vi "Tetra_RX-PROD_Payload.vi"(8 "error in":errorcluster, 10 "Input Constants":string[](array[string]), 11 "Parameters":string[](array[string])=["room", "18.75", "1", "0", "1", "15.5", "31.5"]) -> (0 "error out":errorcluster={"status"=FALSE, "code"=1073676294, "source"="VISA Read in Tetra Loop Serial.vi:4650001->Tetra_Read Imon.vi->Tetra_TX_Payload.vi"}, 2 "Payload Results":string[](array[string])=["0.000", "0.000", "0.000", "0.000", "0.000", "0.000", "0.000", "0.000", "-32.000", "1.000", "18.390", "0.998", "1.810", "3.312", "0.996", "1.198", "5.011", "3.316", "2.513", "2.513", "3.600", "5.496", "2.776", "2.768", "2.280", "1.360", "0.187", "0.089", "0.321", "0.340", "1.483", "0.530", "0.827", "7.000", "P0003", "trace file path"])   [LabVIEW 2018]
uses:
  <vilib>/Utility/error.llb/whitespace.ctl
  86bda725-ccdc-470a-af55-6d3338402ab6.vi
  75c5a050-687e-4f44-8c48-20552f3390b7.vi
  458b4a15-084f-46bd-ad65-8d84519d0715.vi
  e7e3a4d5-9ed6-4285-8f90-f7af1205463a.vi
  778a857b-ea1c-4c41-85f0-8bde546241f8.vi
  765396e5-d7fa-4d1d-a6be-20604e030d46.vi
  498168d9-979f-4171-bbb2-b986919cd012.vi
  fd570da2-80e1-4258-b5ac-03cfe2f2c2d7.vi
  51f53847-2d88-46b1-9baf-ea88b261c08d.vi
  7f90040b-45cf-45e9-9a76-a1a76b3da838.vi
  Initialize References/Station References Global.vi
  Initialize References/Sequence Globals.vi
  Tetra_Globals.vi
  Infrastructure/Test Result File Name Global.vi
  Infrastructure/Test Parameter Globals_1.0.0.vi
  Instruments/Agilent N5232A PNA-L/Labview Driver/Keysight PNA Series/Keysight PNA Series.lvlib
  Instruments/PNA/lib functions/Agilent ENA Series.lvlib
panel:
  out "#of_adc-resyncs":i32
  out "result path":string
  out "ser_rd":string
  out "readback":string
  out "NF_OFS_GHZ":dbl
  out "RX-PASS?(T)":bool
  out "no_fault":bool
  out "FH_NOT(T)":bool
  in  "ess_error":errorcluster
  out "STOP(T)":bool
  in  "Tab Control":enum32{"Page 1", "Page 2", "Page 3", "Page 4"}(tab)
  out "MEAS_DCMON":bool=TRUE
  out "MEAS_ADAR_TEMP":bool
  out "MEAS_PLATE_TEMP":bool
  out "MODE":bool
  out "ADC_ETH(T)":bool
  out "ADC_CAL(t)":bool
  out "ADC_SYNC_NOT":bool
  out "dBFS_REF":dbl
  out "#OFAVGs-Sig":i32
  out "Temp Soak(min)":dbl
  out "NF Freq Out":dbl
  out "RX_GAIN(t)":bool
  out "RX_FILT(t)":bool
  out "RF_POWER(t)":bool
  out "RX_PORT(t)":bool
  out "V_SUPPLY(t)":bool
  out "TEMP(t)":bool
  out "REF_PWR(t)":bool
  out "RF_FREQ(t)":bool
  out "ref_freq(t)":bool
  out "freq/filt change":bool
  out "MEAS_PS":bool=TRUE
  out "GET_TRACE":bool
  out "MEAS_SNR":bool
  out "TEMP":dbl
  out "RX_PORT":i32
  out "REF_POW":dbl=1.0
  out "V_SUPPLY":dbl=18.75
  out "RF_POWER":dbl=6.0
  out "RX_FILT":i32=32
  out "RX_GAIN":i32
  out "RF_FREQ":dbl
  out "GAIN_HSL":dbl
  out "GAIN_LSL":dbl
  out "NF_LSL":dbl
  out "adc_lock(t)":bool
  out "freq_lock(t)":bool
  out "NF_HSL":dbl
  out "RunAM_Init":bool=TRUE
  out "rx_gain_auto(t)":bool
  out "rdiv(v)":dbl[](array[numeric])=[3.6, 5.496, 2.776, 2.768, 2.28, 1.36]
  out "rdiv(i)":dbl[](array[numeric])=[0.187, 0.089, 0.321, 0.34, 1.483, 0.53]
  out "rdv":dbl[](array[numeric])=[18.39, 0.998, 1.81, 3.312, 0.996, 1.198, 5.011, 3.316, 2.513, 2.513]
  out "temp_sense1-2":dbl[](array[numeric])
  out "ob_temp":sgl[](array[numeric])
  out "ps_meas(i)(w)":dbl[](array[numeric])
  out "rxgain (1-4)":i32[](array[numeric])
  out "rxpeak_mhz":dbl
  out "rxpeak_dbm":dbl
  out "fout_bp":dbl
  out "rx_bpower_on":dbl
  out "rx_bpower_off":dbl
  out "BW(MHz)":dbl
  out "rx_filt":i32
  out "bpf":i32=1
  out "noisecapture path":string
  out "sigcapture path":string
  out "TraceFilePath":path
  out "DC_LSL":dbl
  out "DC_HSL":dbl
  out "cal_rf_ampl":dbl
  out "cal_ref_ampl":dbl
  out "cal_ref_freq":dbl
  out "cal_rf_freq":dbl
  out "peak_gain":dbl
  out "s-n":dbl
  out "nf":dbl
  out "if_freq":dbl
  out "ref_freq":dbl
  out "Cutoff Freq (GHz)":dbl
  out "adc#ofresync":i32
  out "cal_adc_delay":string
  out "comport":refnum<visa-resource-name>
  out "CalFileA":path
  out "adc_chan_id":string
  out "relative seconds":dbl=73640.4138221 format="%_19f"
  out "ref_cal":dbl[][](array[numeric])
  out "rf_cal":dbl[][](array[numeric])
  out "iteration Time(s)":dbl
  out "#OFAVGs-Noi":i32
  out "NF_MASK":dbl[][](array[numeric])
  out "adcsync":string="rd rxm 0x31\r\n0x031: 0x67\r\n>"
  # "Globals (last value change)"
  # "Vmon & Imon"
  # "Temp Sensors"
types:
  T1 = typedef "whitespace.ctl" = u16
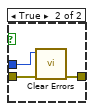
[diagram p3: hidden frame]
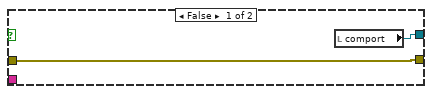
[diagram p4: hidden frame]
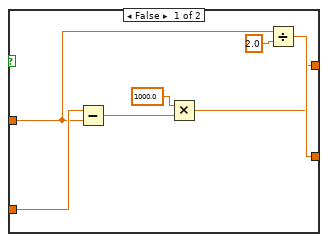
[diagram p5: hidden frame]
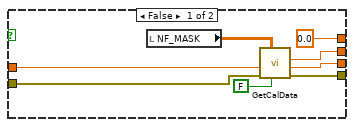
[diagram p7: hidden frame]
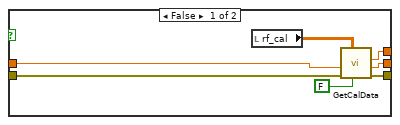
[diagram p8: hidden frame]
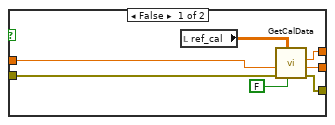
[diagram p9: hidden frame]
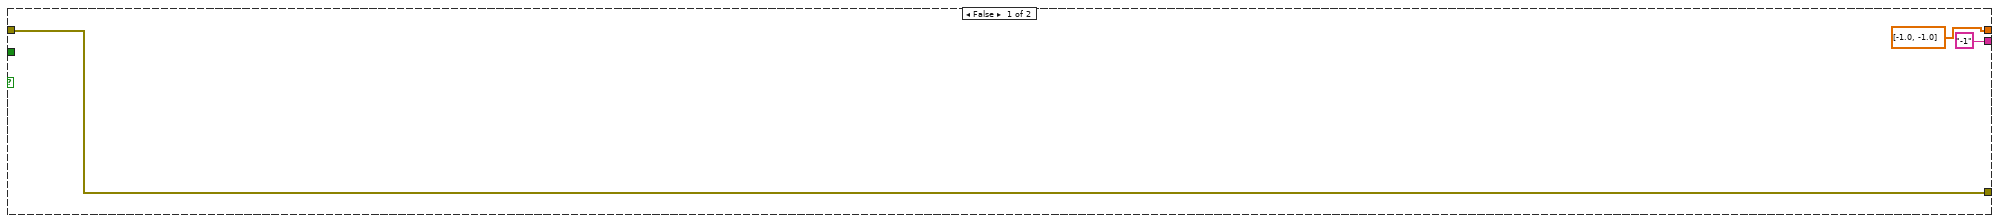
[diagram p11: hidden frame]
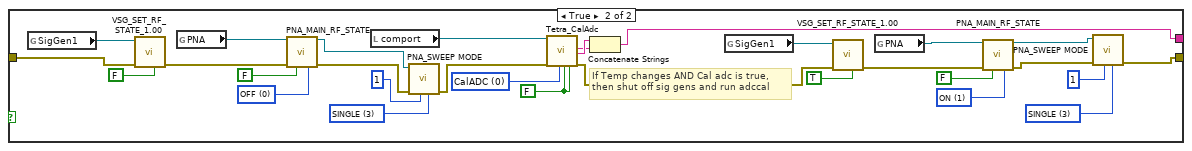
[diagram p12: hidden frame]
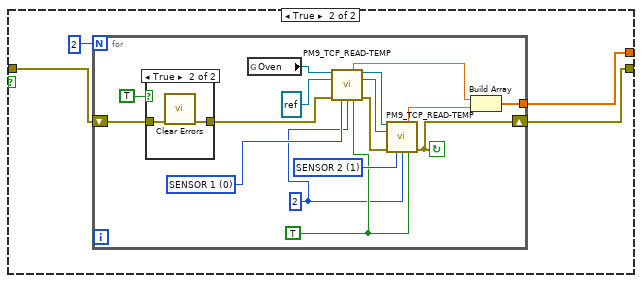
[diagram p13: hidden frame]
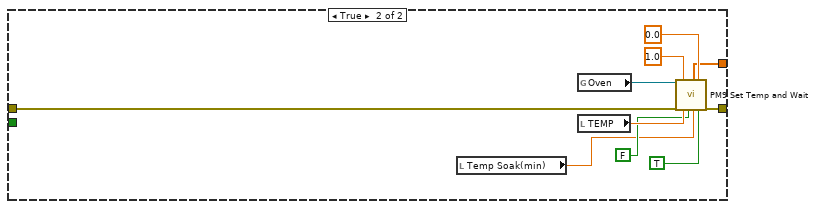
[diagram p15: hidden frame]
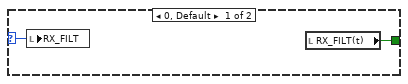
[diagram p16: hidden frame]
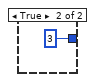
[diagram p17: hidden frame]
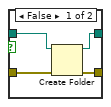
[diagram p19: hidden frame]
diagram:
  n1 = flat-sequence {
    tunnel: [w30] -> w19
    tunnel: [w31] -> w15
    tunnel: "error in" -> [w30]
    tunnel: [w68] -> w29
    tunnel: [w67] -> w28
    tunnel: [w66] -> w27
    tunnel: [w65] -> w26
    tunnel: [w64] -> w25
    tunnel: [w63] -> w24
    tunnel: [w62] -> w23
    tunnel: [w61] -> w22
    tunnel: [w60] -> w21
    tunnel: [w59] -> w20
    tunnel: w19 -> [w58]
    tunnel: [w57] -> w18
    tunnel: [w56] -> w16
    tunnel: w15 -> [w53]
    tunnel: w29 -> [w1117]
    tunnel: w28 -> [w1116]
    tunnel: w27 -> [w1115]
    tunnel: w26 -> [w1114]
    tunnel: w25 -> [w1113]
    tunnel: w24 -> [w1112]
    tunnel: w23 -> [w1111]
    tunnel: w22 -> [w1110]
    tunnel: w21 -> [w1109]
    tunnel: w20 -> [w1108]
    tunnel: w18 -> [w1106]
    tunnel: w16 -> [w1105]
    tunnel: [w1117] -> w13
    tunnel: [w1116] -> w12
    tunnel: [w1115] -> w11
    tunnel: [w1114] -> w10
    tunnel: [w1113] -> w9
    tunnel: [w1112] -> w8
    tunnel: [w1111] -> w7
    tunnel: [w1110] -> w6
    tunnel: [w1109] -> w5
    tunnel: [w1108] -> w4
    tunnel: [w1107] -> w3
    tunnel: [w1106] -> w2
    tunnel: [w1102] -> w1
    tunnel: [w1199] -> w17
    tunnel: w13 -> [w1187]
    tunnel: w12 -> [w1188]
    tunnel: w11 -> [w1189]
    tunnel: w10 -> [w1190]
    tunnel: w9 -> [w1185]
    tunnel: w8 -> [w1184]
    tunnel: w7 -> [w1183]
    tunnel: w6 -> [w1182]
    tunnel: w5 -> [w1186]
    tunnel: w4 -> [w1194]
    tunnel: w3 -> [w1181]
    tunnel: w2 -> [w1199]
    tunnel: w1 -> [w1180]
    frame #0 {
      n2 = flat-sequence {
        frame #0 {
          w49 = TRUE ("Test Running (T)")
          n3 = global read "Station References Global.vi" "Gantry"() -> (w50:refnum<visa-resource-name>)
          n4 = call "WAM_ESS.vi"("VISA resource name"=w50, "error in (no error)"="ess_error", "Open Serial"=w49, "Test Running (T)"=w49, "Close Serial"=w49) -> ("FH_NOT(T)"=→"FH_NOT(T)":bool, "error out"=w47:errorcluster)  [unwired: 7 in, 2 out]
          n5 = local write "ess_error"(w47) -> ()
        }
      }
      n6 = call <vilib>:"High Resolution Relative Seconds.vi"() -> ("relative seconds"=→"relative seconds":dbl)
      n7 = First Call?() -> (First Call?: T/F=w32:bool)
      n8 = case shown="True" w32 {
        frame False {
        }
        frame True {
          (unwired) path "C:/3500007_TetraFinalTestAnalysis/testreport.ini" ("*.ini file")
          n9 = global read "Tetra_Globals.vi" "comport"() -> (w38:refnum<visa-resource-name>)
          n10 = VISA Close(VISA resource name=w38) -> ()  [unwired: 1 in, 1 out]
          n11 = global read "Sequence Globals.vi" "DevSupportPath"() -> (w41:path)
          n12 = global read "Tetra_Globals.vi" "RevC(t)"() -> (w37:bool)
          n13 = global read "Test Result File Name Global.vi" "Test Results File Name"() -> (w36:path)
          n14 = global read "Sequence Globals.vi" "AppSupportPath 2"() -> (w43:path)
          n15 = Not(x=w37) -> ()  [unwired: 1 out]
          n16 = Build Path(base path=w41, name or relative path=path "3500007_TetraFinalTestAnalysis/testreport.ini" ("*.ini file")) -> (appended path=w39:path)
          n17 = Strip Path(path=w39) -> (name=w45:string)  [unwired: 1 out]
          n18 = global read "Sequence Globals.vi" "IsRuntime?"() -> (w44:bool)
          n19 = Build Path(base path=w43, name or relative path=w45) -> (appended path=w42:path)
          n20 = Path To String(path=w36) -> (string=→"result path":string)
          n21 = Select(t=w42, s=w44, f=w39) -> (s? t:f=w46:path)
          n22 = call "ProdLimits.vi"("*.ini file"=w46) -> ()  [unwired: 9 in, 2 out]
          "RunAM_Init" <- TRUE ("RunAM_Init")
        }
      }
      n23 = global read "Sequence Globals.vi" "Stop Testing"() -> (w31:bool)
    }
    frame #1 {
      n24 = Select(t=0, s=w53, f=2) -> (s? t:f=w54:i32)
      n25 = for {
        N: w54 -> [_]
        tunnel: [w95] -> w68
        tunnel: [w94] -> w67
        tunnel: [w93] -> w60
        tunnel: [w92] -> w66
        tunnel: [w91] -> w65
        tunnel: [w90] -> w59
        tunnel: [w89] -> w64
        tunnel: [w88] -> w63
        tunnel: [w87] -> w62
        tunnel: [w86] -> w61
        tunnel: w58 -> [w85]
        shift-right: [w78] -> w57
        shift-left: _ -> [_]
        tunnel: [w72] -> w56 mode=indexing
        i -> [w75]
        stop <- w81 stop-if-true
        n26 = flat-sequence {
          tunnel: [w127] -> w122
          tunnel: ["Parameters"] -> w121
          tunnel: ["Input Constants"] -> w120
          tunnel: w85 -> [w127]
          tunnel: w122 -> [w142]
          tunnel: [w141] -> w119
          tunnel: w121 -> [w212]
          tunnel: w120 -> [w211]
          tunnel: [w203] -> w118
          tunnel: [w199] -> w117
          tunnel: [w210] -> w116
          tunnel: [w209] -> w115
          tunnel: [w208] -> w114
          tunnel: [w187] -> w113
          tunnel: [w207] -> w112
          tunnel: [w200] -> w111
          tunnel: [w189] -> w110
          tunnel: [w161] -> w109
          tunnel: [w175] -> w108
          tunnel: [FALSE] -> w69
          tunnel: w119 -> [w292]
          tunnel: [w292] -> w107
          tunnel: w118 -> [w265]
          tunnel: w117 -> [w289]
          tunnel: w116 -> [w287]
          tunnel: w115 -> [w286]
          tunnel: w114 -> [w284]
          tunnel: w113 -> [w282]
          tunnel: w112 -> [w280]
          tunnel: w111 -> [w276]
          tunnel: w110 -> [w277]
          tunnel: w109 -> [w274]
          tunnel: w108 -> [w271]
          tunnel: w69 -> [w262]
          tunnel: w107 -> [w300]
          tunnel: [w301] -> w106
          tunnel: w106 -> [w366]
          tunnel: [w366] -> w105
          tunnel: [w392] -> w104
          tunnel: w105 -> [w393]
          tunnel: w104 -> [w483]
          tunnel: [w483] -> w103
          tunnel: [w494] -> w82
          tunnel: w103 -> [w493]
          tunnel: [w535] -> w102
          tunnel: w82 -> [w532]
          tunnel: w102 -> [w544]
          tunnel: [w545] -> w101
          tunnel: w101 -> [w564]
          tunnel: [w556] -> w100
          tunnel: w100 -> [w615]
          tunnel: [w614] -> w99
          tunnel: [w705] -> w98
          tunnel: w99 -> [w704]
          tunnel: w98 -> [w726]
          tunnel: [w721] -> w97
          tunnel: w97 -> [w959]
          tunnel: [w958] -> w96
          tunnel: w96 -> [w980]
          tunnel: [w982] -> w84
          tunnel: w84 -> [w1008]
          tunnel: [w1008] -> w71
          tunnel: [w1007] -> w83
          tunnel: w71 -> [w1035]
          tunnel: [w1035] -> w70
          tunnel: [w1048] -> w77
          tunnel: [w1087] -> w95
          tunnel: [w1078] -> w94
          tunnel: [w1082] -> w93
          tunnel: [w1071] -> w92
          tunnel: [w1068] -> w91
          tunnel: [w1063] -> w90
          tunnel: [w1058] -> w89
          tunnel: [w1056] -> w88
          tunnel: [w1053] -> w87
          tunnel: [w1050] -> w86
          tunnel: w70 -> [w1048]
          frame #0 {
          }
          frame #1 {
            n27 = Index Array(array=w211, index #1=2 ("index"), index #2=5 ("index"), index #3=3 ("index"), index #4=6 ("index"), index #6=10 ("index"), index #7=15 ("index"), index #8=13 ("index"), index #9=11 ("index"), index #10=8 ("index"), index #12=18 ("index"), index #13=20 ("index"), index #17=26 ("index")) -> (element #1=w144:string, element #2=w171:string, element #3=w177:string, element #4=w227:string, element #5=w226:string, element #6=w217:string, element #7=w214:string, element #8=w139:string, element #9=w197:string, element #10=w178:string, element #11=w183:string, element #12=w152:string, element #13=w162:string, element #14=w160:string, element #15=w158:string, element #16=w156:string, element #17=→"ser_rd":string)  [unwired: 5 in]
            n28 = call "StringToNumberControlWithBool.vi"("String In"=w177) -> ("NOT = 0"=→"MODE":bool)  [unwired: 7 in, 1 out]
            n29 = call "StringToNumberControlWithBool.vi"("String In"=w227) -> ("Number Out"=→"Temp Soak(min)":dbl)  [unwired: 7 in, 1 out]
            n30 = call "StringToNumberControlWithBool.vi"("String In"=w217) -> ("NOT = 0"=→"GET_TRACE":bool)  [unwired: 7 in, 1 out]
            n31 = Fract/Exp String To Number(string=w197) -> (number=→"Cutoff Freq (GHz)":dbl)  [unwired: 3 in, 1 out]
            n32 = call "StringToNumberControlWithBool.vi"("String In"=w162) -> ("NOT = 0"=→"ADC_CAL(t)":bool)  [unwired: 7 in, 1 out]
            n33 = Fract/Exp String To Number(string=w160) -> (number=→"dBFS_REF":dbl)  [unwired: 3 in, 1 out]
            n34 = String To Path(string=w214) -> (path=→"CalFileA":path)
            n35 = Match Pattern(string=w226, regular expression=";") -> (before substring=w225:string, after substring=w224:string)  [unwired: 1 in, 2 out]
            n36 = call "StringToNumberControlWithBool(x2).vi"("Seperator"=";", "string"=w139) -> ("Num"=→"#OFAVGs-Sig":dbl, "after substring"=w137:string, "Seperator Out"=w134:string)  [unwired: 3 in, 4 out]
            n37 = Match Pattern(string=w178, regular expression=";") -> (before substring=w193:string, after substring=w191:string)  [unwired: 1 in, 2 out]
            n38 = Match Pattern(string=w171, regular expression=";") -> (before substring=w173:string, after substring=w170:string)  [unwired: 1 in, 2 out]
            n39 = Match Pattern(string=w183, regular expression=";") -> (before substring=w182:string, after substring=w181:string)  [unwired: 1 in, 2 out]
            n40 = call "StringToNumberControlWithBool(x2).vi"("Seperator"=";", "string"=w152) -> ("Num(2)"=→"#of_adc-resyncs":dbl, "NOT_0(2)"=w151:bool, "NOT_0?"=→"ADC_ETH(T)":bool, "Seperator Out"=w155:string)  [unwired: 3 in, 3 out]
            n41 = First Call?() -> (First Call?: T/F=w143:bool)
            n42 = Not(x=w151) -> (.not. x?=→"ADC_SYNC_NOT":bool)
            n43 = case shown="True" w143 {
              tunnel: [w231 w237] -> w145
              tunnel: w144 -> [_ w239]
              tunnel: w142 -> [w230 w232]
              tunnel: [w230 w236] -> w141
              frame False {
                n44 = local read "comport"() -> (w231:refnum<visa-resource-name>)
              }
              frame True {
                n45 = Empty String/Path?(string/path=w239) -> (empty?=w240:bool)
                n46 = global read "Tetra_Globals.vi" "comport"() -> (w234:refnum<visa-resource-name>)
                n47 = Select(t=w234, s=w240, f=w239) -> (s? t:f=w238:refnum<visa-resource-name>)
                n48 = call "Tetra Serial.vi"("COMPORT"=w238, "ClearErrorIn(t)"=TRUE, "error in (no error)"=w232, "Open Ser(t)"=TRUE) -> ("comport"=w237:refnum<visa-resource-name>, "error out"=w236:errorcluster)  [unwired: 7 in, 3 out]
              }
            }
            "comport" <- w145
            n49 = call "StringToNumberControlWithBool.vi"("String In"=w225) -> ("NOT = 0"=→"MEAS_PS":bool)  [unwired: 7 in, 1 out]
            n50 = call "StringToNumberControlWithBool.vi"("String In"=w224) -> ("NOT = 0"=→"MEAS_DCMON":bool)  [unwired: 7 in, 1 out]
            n51 = call "StringToNumberControlWithBool(x2).vi"("Seperator"=w134, "string"=w137) -> ("Num(2)"=→"NF_OFS_GHZ":dbl, "Num"=→"#OFAVGs-Noi":dbl)  [unwired: 3 in, 5 out]
            n52 = call "StringToNumberControlWithBool.vi"("String In"=w193) -> ("NOT = 0"=w175:bool)  [unwired: 7 in, 1 out]
            "MEAS_SNR" <- w175
            n53 = call "StringToNumberControlWithBool.vi"("String In"=w191) -> ("Number Out"=→"BW(MHz)":dbl)  [unwired: 7 in, 1 out]
            n54 = Fract/Exp String To Number(string=w170) -> (number=w169:dbl)  [unwired: 3 in, 1 out]
            n55 = Index Array(array=w212) -> (element #1=w187:string, element #2=w220:string, element #3=w219:string, element #4=w206:string, element #5=w205:string, element #6=w195:string, element #7=w204:string, element #8=w202:string)  [unwired: 8 in]
            n56 = call "StringToNumberControlWithBool.vi"("String In"=w182) -> ("NOT = 0"=→"MEAS_ADAR_TEMP":bool)  [unwired: 7 in, 1 out]
            n57 = call "StringToNumberControlWithBool.vi"("String In"=w181) -> ("NOT = 0"=→"MEAS_PLATE_TEMP":bool)  [unwired: 7 in, 1 out]
            n58 = call "StringToNumberControlWithBool(x2).vi"("Seperator"=w155, "string"=w158) -> ("Num(2)"=→"DC_HSL":dbl, "Num"=→"DC_LSL":dbl, "Seperator Out"=w157:string)  [unwired: 3 in, 4 out]
            n59 = Equal?(x=w173, y="fixed") -> (x = y?=w168:bool)
            n60 = call "StringToNumberControlWithBool(x2).vi"("Seperator"=w157, "string"=w156) -> ("Num(2)"=→"GAIN_HSL":dbl, "Num"=→"GAIN_LSL":dbl)  [unwired: 3 in, 5 out]
            n61 = Fract/Exp String To Number(string=w220) -> (number=w208:dbl)  [unwired: 3 in, 1 out]
            "V_SUPPLY" <- w208
            n62 = Decimal String To Number(string=w219) -> (number=w209:i32)  [unwired: 2 in, 1 out]
            "RX_PORT" <- w209
            n63 = Fract/Exp String To Number(string=w206) -> (number=w207:dbl)  [unwired: 3 in, 1 out]
            "REF_POW" <- w207
            n64 = Fract/Exp String To Number(string=w205) -> (number=w210:dbl)  [unwired: 3 in, 1 out]
            "RF_POWER" <- w210
            n65 = Decimal String To Number(string=w195) -> (number=w199:i32)  [unwired: 2 in, 1 out]
            "RX_FILT" <- w199
            n66 = Decimal String To Number(string=w204) -> (number=w203:i32)  [unwired: 2 in, 1 out]
            "RX_GAIN" <- w203
            n67 = call "TempControlWithBool.vi"("INPUT"=w187) -> ("out"=→"TEMP":dbl, "Valid(t)"=w161:bool)  [unwired: 6 in, 1 out]
            n68 = Fract/Exp String To Number(string=w202) -> (number=w200:dbl)  [unwired: 3 in, 1 out]
            "RF_FREQ" <- w200
            n69 = case "calculate the if and ref" shown="True" w168 {
              tunnel: w200 -> [w245 w257]
              tunnel: [w246 w256] -> w189
              tunnel: [w242 w255] -> w188
              tunnel: w169 -> [w244 w248]
              frame False {
                n70 = Subtract(x=w245, y=w244) -> (x-y=w243:dbl)
                n71 = Multiply(x=1000.0, y=w243) -> (x*y=w242:dbl)
                n72 = Divide(x=w244, y=2.0) -> (x/y=w246:dbl)
              }
              frame True {
                w250 = 2.0 ("y")
                n73 = Less Than 0?(x=w248) -> (x < 0?=w249:bool)
                n74 = Divide(x=w248, y=1000.0) -> (x/y=w253:dbl)
                n75 = case shown="True" w249 {
                  tunnel: [w258 w261] -> w255
                  tunnel: w248 -> [w258 w260]
                  frame False {
                  }
                  frame True {
                    n76 = Multiply(x=w260, y=-1.0) -> (x*y=w261:dbl)
                  }
                }
                n77 = Divide(x=w253, y=w250) -> (x/y=w251:dbl)
                n78 = Divide(x=w257, y=w250) -> (x/y=w252:dbl)
                n79 = Add(x=w252, y=w251) -> (x+y=w256:dbl)
              }
            }
            "ref_freq" <- w189
            "if_freq" <- w188
            n80 = global write "Tetra_Globals.vi" "TEMP(t)"(w161) -> ()
          }
          frame #2 {
            # "Check if value changed\nif value changed (t) use to skip the routine"
            n81 = Stop(stop? (T)=w262) -> ()
            n82 = global read "Tetra_Globals.vi" "RX_N_FREQ_LIST"() -> (w269:dbl[])
            n83 = call "Is Value Changed.vim"("value"=w282) -> ("changed or first call?"=w283:bool)
            n84 = call "Is Value Changed.vim"("value"=w277) -> ("changed or first call?"=→"ref_freq(t)":bool)
            n85 = call "Is Value Changed.vim"("value"=w284) -> ("changed or first call?"=→"V_SUPPLY(t)":bool)
            n86 = call "Is Value Changed.vim"("value"=w286) -> ("changed or first call?"=→"RX_PORT(t)":bool)
            n87 = call "Is Value Changed.vim"("value"=w280) -> ("changed or first call?"=→"REF_PWR(t)":bool)
            n88 = call "Is Value Changed.vim"("value"=w287) -> ("changed or first call?"=→"RF_POWER(t)":bool)
            n89 = call "Is Value Changed.vim"("value"=w289) -> ("changed or first call?"=→"RX_FILT(t)":bool)
            n90 = call "Is Value Changed.vim"("value"=w265) -> ("changed or first call?"=→"RX_GAIN(t)":bool)
            n91 = call "Is Value Changed.vim"("value"=w276) -> ("changed or first call?"=→"RF_FREQ(t)":bool)
            n92 = Equal?(x=w265, y=-1) -> (x = y?=→"rx_gain_auto(t)":bool)
            n93 = And(x=w283, y=w274) -> (x .and. y?=→"TEMP(t)":bool)
            n94 = Empty Array?(array=w269) -> (empty?=w267:bool)
            n95 = Array Size(array=w269) -> (size(s)=w273:i32)
            n96 = for {
              tunnel: w269 -> [w299] mode=indexing
              tunnel: [w297] -> w272
              tunnel: w273 -> [w293]
              i -> [w294]
              stop <- w296 stop-if-true
              n97 = local read "RF_FREQ"() -> (w298:dbl)
              n98 = Equal?(x=w293, y=w294) -> (x = y?=w295:bool)
              n99 = Equal?(x=w299, y=w298) -> (x = y?=w297:bool)
              n100 = Or(x=w297, y=w295) -> (x .or. y?=w296:bool)
            }
            n101 = And(x=w272, y=w271) -> (x .and. y?=w270:bool)
            n102 = Or(x=w267, y=w270) -> (x .or. y?=w268:bool)
            n103 = local write "MEAS_SNR"(w268) -> ()
          }
          frame #3 {
            n104 = flat-sequence {
              tunnel: w300 -> [w317]
              tunnel: [w304] -> w301
              frame #0 {
                n105 = local read "ref_freq"() -> (w312:dbl)
                n106 = Multiply(x=1000.0, y=w312) -> (x*y=w310:dbl)
                n107 = First Call?() -> (First Call?: T/F=w309:bool)
                n108 = case shown="True" w309 {
                  tunnel: [w355 w364] -> w319
                  tunnel: [w354 w363] -> w318
                  tunnel: w317 -> [w353 w361]
                  tunnel: [w352 w360] -> w316
                  tunnel: w310 -> [w351 w358]
                  frame False {
                    n109 = local read "ref_cal"() -> (w357:dbl[][])
                    n110 = call "GetCalData.vi"("Open new file T"=FALSE, "Ary In"=w357, "error in (no error)"=w353, "RF Freq (MHz)"=w351) -> ("error out"=w352:errorcluster, "Ampl Out"=w354:dbl, "Cal Freq Out"=w355:dbl)  [unwired: 2 in, 3 out]
                  }
                  frame True {
                    n111 = global read "Tetra_Globals.vi" "REF_CAL"() -> (w365:dbl[][])
                    n112 = call "GetCalData.vi"("Open new file T"=FALSE, "Ary In"=w365, "error in (no error)"=w361, "RF Freq (MHz)"=w358) -> ("error out"=w360:errorcluster, "Ampl Out"=w363:dbl, "Cal Freq Out"=w364:dbl, "array out"=→"ref_cal":dbl[][])  [unwired: 2 in, 2 out]
                  }
                }
                "cal_ref_freq" <- w319
                "cal_ref_ampl" <- w318
                n113 = local read "RF_FREQ"() -> (w302:dbl)
                n114 = Multiply(x=1000.0, y=w302) -> (x*y=w308:dbl)
                n115 = case shown="True" w309 {
                  tunnel: [w340 w349] -> w315
                  tunnel: [w339 w348] -> w314
                  tunnel: w316 -> [w338 w346]
                  tunnel: [w337 w345] -> w305
                  tunnel: w308 -> [w336 w343]
                  frame False {
                    n116 = local read "rf_cal"() -> (w342:dbl[][])
                    n117 = call "GetCalData.vi"("Open new file T"=FALSE, "Ary In"=w342, "error in (no error)"=w338, "RF Freq (MHz)"=w336) -> ("error out"=w337:errorcluster, "Ampl Out"=w339:dbl, "Cal Freq Out"=w340:dbl)  [unwired: 2 in, 3 out]
                  }
                  frame True {
                    n118 = global read "Tetra_Globals.vi" "RX_INPUT_OFFSET"() -> (w350:dbl[][])
                    n119 = call "GetCalData.vi"("Open new file T"=FALSE, "Ary In"=w350, "error in (no error)"=w346, "RF Freq (MHz)"=w343) -> ("error out"=w345:errorcluster, "Ampl Out"=w348:dbl, "Cal Freq Out"=w349:dbl, "array out"=→"rf_cal":dbl[][])  [unwired: 2 in, 2 out]
                  }
                }
                "cal_rf_freq" <- w315
                "cal_rf_ampl" <- w314
                n120 = case shown="True" w309 {
                  tunnel: w302 -> [w327 w334]
                  tunnel: [w326 w333] -> w307
                  tunnel: [0.0 ("NF_LSL") 0.0 ("NF_LSL")] -> w306
                  tunnel: w305 -> [w322 w329]
                  tunnel: [w321 w330] -> w304
                  tunnel: [w320 w328] -> w303
                  frame False {
                    n121 = local read "NF_MASK"() -> (w324:dbl[][])
                    n122 = call "GetCalData.vi"("Open new file T"=FALSE, "Ary In"=w324, "error in (no error)"=w322, "RF Freq (MHz)"=w327) -> ("error out"=w321:errorcluster, "Ampl Out"=w326:dbl, "Cal Freq Out"=w320:dbl)  [unwired: 2 in, 3 out]
                  }
                  frame True {
                    n123 = global read "Tetra_Globals.vi" "NF_MASK"() -> (w335:dbl[][])
                    "NF_MASK" <- w335
                    n124 = call "GetCalData.vi"("Open new file T"=FALSE, "Ary In"=w335, "error in (no error)"=w329, "RF Freq (MHz)"=w334) -> ("error out"=w330:errorcluster, "Ampl Out"=w333:dbl, "Cal Freq Out"=w328:dbl)  [unwired: 2 in, 3 out]
                  }
                }
                "NF_LSL" <- w306
                "NF_HSL" <- w307
                "NF Freq Out" <- w303
              }
            }
          }
          frame #4 {
            n125 = flat-sequence {
              frame #0 {
                n126 = local read "RX_PORT(t)"() -> (w371:bool)
                n127 = local read "ess_error"() -> (w368:errorcluster)
                n128 = And(x=TRUE, y=w371) -> (x .and. y?=w370:bool)
                n129 = case shown="True" w370 {
                  tunnel: w368 -> [w372 w382]
                  tunnel: [w372 w381] -> w367
                  frame False {
                  }
                  frame True {
                    w378 = u16 0 items=["Inches", "cm"] ("Zunits")
                    # "convert to Gantry location"
                    n130 = local read "RX_PORT"() -> (w374:i32)
                    n131 = global read "Tetra_Globals.vi" "Gantry_Z"() -> (w376:dbl)
                    n132 = global read "Station References Global.vi" "Gantry"() -> (w379:refnum<visa-resource-name>)
                    n133 = Subtract(x=21, y=w374) -> (x-y=w373:i32)
                    n134 = call "Gantry.vi"("COMPORT"=w379, "error in (no error)"=w382, "Antenna Select"=w373, "z ref"=21.0, "Write(reads antenna co-ords when off)"=TRUE, "z"=w376, "Zunits"=w378) -> ("error out"=w381:errorcluster)  [unwired: 12 in]
                  }
                }
                n135 = local write "ess_error"(w367) -> ()
              }
            }
          }
          frame #5 {
            n136 = local read "RX_PORT(t)"() -> (w383:bool)
            n137 = local read "MEAS_PLATE_TEMP"() -> (w387:bool)
            n138 = global read "Tetra_Globals.vi" "TEMP(t)"() -> (w390:bool)
            n139 = First Call?() -> (First Call?: T/F=w385:bool)
            n140 = Or(x=w383, y=w385) -> (x .or. y?=w384:bool)
            n141 = Or(x=w390, y=w387) -> (x .or. y?=w389:bool)
            n142 = Or(x=w387, y=w384) -> (x .or. y?=w386:bool)
            n143 = case shown="True" w389 {
              tunnel: w393 -> [w395 w409]
              tunnel: [w395 w403] -> w392
              tunnel: [sgl[] [-1.0, -1.0] ("temp") w408] -> w391
              tunnel: ["-1" ("cal_adc_delay") w400] -> w388
              tunnel: w386 -> [_ w398]
              frame False {
              }
              frame True {
                n144 = global read "Station References Global.vi" "Oven Present?"() -> (w397:bool)
                n145 = local read "ADC_CAL(t)"() -> (w405:bool)
                n146 = local read "TEMP(t)"() -> (w407:bool)
                n147 = And(x=w398, y=w397) -> (x .and. y?=w399:bool)
                n148 = And(x=w407, y=w405) -> (x .and. y?=w406:bool)
                n149 = case shown="False" w407 {
                  tunnel: w409 -> [w445 w477]
                  tunnel: [w443 w476] -> w404
                  tunnel: [w444 w474] -> w408
                  tunnel: w399 -> [w442 _]
                  frame False {
                    n150 = case shown="False" w442 {
                      tunnel: w445 -> [w446 w451]
                      tunnel: [sgl[] [-1.0, -1.0] w450] -> w444
                      tunnel: [w446 w449] -> w443
                      frame False {
                      }
                      frame True {
                        n151 = for {
                          N: 2 -> [_]
                          tunnel: [w462] -> w450
                          shift-right: [w458] -> w449
                          shift-left: w451 -> [w456]
                          stop <- w458 continue-if-true
                          w452 = u32 2 ("milliseconds to wait")
                          w454 = TRUE ("Close tcp(t)")
                          w460 = u16 1 items=["SENSOR 1", "SENSOR 2"] ("Sensor")
                          w461 = u16 0 items=["SENSOR 1", "SENSOR 2"] ("Sensor")
                          n152 = case shown="True" TRUE {
                            tunnel: [w468 w470] -> w457
                            tunnel: w456 -> [w468 w469]
                            frame False {
                            }
                            frame True {
                              n153 = call <vilib>:"Clear Errors.vi"("error in (no error)"=w469) -> ("error out"=w470:errorcluster)  [unwired: 5 in, 1 out]
                            }
                          }
                          n154 = global read "Station References Global.vi" "Oven"() -> (w467:refnum<visa-resource-name>)
                          n155 = call "PM9_TCP_READ-TEMP.vi"("VISA"=w467, "connection ID"=refnum<k5> refnum, "error in (no error)"=w457, "Sensor"=w461, "milliseconds to wait"=w452, "Close tcp(t)"=w454) -> ("Value"=w463:sgl, "visa out"=w459:refnum<visa-resource-name>, "connection ID out"=w466:refnum<k5>, "error out"=w465:errorcluster)  [unwired: 6 in]
                          n156 = call "PM9_TCP_READ-TEMP.vi"("VISA"=w459, "connection ID"=w466, "error in (no error)"=w465, "Sensor"=w460, "milliseconds to wait"=w452, "Close tcp(t)"=w454) -> ("Value"=w464:sgl, "error out"=w458:errorcluster)  [unwired: 6 in, 2 out]
                          n157 = Build Array(w463, w464) -> (w462:sgl[])
                        }
                      }
                    }
                  }
                  frame True {
                    n158 = local read "Temp Soak(min)"() -> (w471:dbl)
                    n159 = global read "Station References Global.vi" "Oven"() -> (w475:refnum<visa-resource-name>)
                    n160 = local read "TEMP"() -> (w473:dbl)
                    n161 = call "PM9 Set Temp and Wait.vi"("VISA"=w475, "Error In"=w477, "Accuracy +/-"=1.0, "Set Point"=w473, "RO(t)"=FALSE, "Min (-1 for cont.)"=w471, "Refresh Rate(s)"=0.0, "close session(t)"=TRUE) -> ("temp"=w474:sgl[], "error out"=w476:errorcluster)  [unwired: 8 in, 2 out]
                  }
                }
                n162 = And(x=FALSE, y=w406) -> (x .and. y?=w402:bool)
                n163 = case shown="False" w402 {
                  tunnel: w404 -> [w411 w440]
                  tunnel: ["-1" ("cal_adc_delay") w415] -> w400
                  tunnel: [w411 w419] -> w403
                  frame False {
                  }
                  frame True {
                    w414 = FALSE ("Open Ser(t)")
                    w418 = 0 items=["CalADC", "ReadADC"] ("ADC_Cal_Function")
                    w431 = 3 items=["HOLD", "CONT", "GROUP", "SINGLE"] ("Mode")
                    w429 = 1 items=["OFF", "ON"] ("STATE(0=OFF)")
                    w432 = 3 items=["HOLD", "CONT", "GROUP", "SINGLE"] ("Mode")
                    w434 = 0 items=["OFF", "ON"] ("STATE(0=OFF)")
                    # "If Temp changes AND Cal adc is true, \nthen shut off sig gens and run adccal"
                    n164 = global read "Station References Global.vi" "SigGen1"() -> (w441:refnum<visa-resource-name>)
                    n165 = call "VSG_SET_RF_STATE_1.00.vi"("RF ON/OFF (OFF)"=FALSE ("Enable RF Power (T: Enable)"), "error in"=w440, "Session In"=w441) -> ("error out"=w439:errorcluster)  [unwired: 6 in, 2 out]
                    n166 = global read "Station References Global.vi" "PNA"() -> (w438:refnum<visa-resource-name>)
                    n167 = call "PNA_MAIN_RF_STATE.vi"("Session In"=w438, "error in"=w439, "RO(T)"=FALSE, "STATE(0=OFF)"=w434) -> ("Session Out"=w437:refnum<visa-resource-name>, "error out"=w436:errorcluster)  [unwired: 9 in, 1 out]
                    n168 = local read "comport"() -> (w413:refnum<visa-resource-name>)
                    n169 = call "PNA_SWEEP MODE.vi"("Mode"=w432, "Channel"=1, "error in (no error)"=w436, "VISA resource name"=w437) -> ("error out"=w412:errorcluster)  [unwired: 6 in, 1 out]
                    n170 = call "Tetra_CalAdc.vi"("COMPORT"=w413, "error in (no error)"=w412, "ADC_Cal_Function"=w418, "Open Ser(t)"=w414, "Close Ser(t)"=w414) -> ("cal_adc_mag"=w416:string, "cal_adc_delay"=w417:string, "error out"=w422:errorcluster)  [unwired: 9 in, 3 out]
                    n171 = Concatenate Strings(w417, w416) -> (w415:string)
                    n172 = global read "Station References Global.vi" "SigGen1"() -> (w423:refnum<visa-resource-name>)
                    n173 = call "VSG_SET_RF_STATE_1.00.vi"("RF ON/OFF (OFF)"=TRUE ("Enable RF Power (T: Enable)"), "error in"=w422, "Session In"=w423) -> ("error out"=w424:errorcluster)  [unwired: 6 in, 2 out]
                    n174 = global read "Station References Global.vi" "PNA"() -> (w425:refnum<visa-resource-name>)
                    n175 = call "PNA_MAIN_RF_STATE.vi"("Session In"=w425, "error in"=w424, "RO(T)"=FALSE, "STATE(0=OFF)"=w429) -> ("Session Out"=w426:refnum<visa-resource-name>, "error out"=w427:errorcluster)  [unwired: 9 in, 1 out]
                    n176 = call "PNA_SWEEP MODE.vi"("Mode"=w431, "Channel"=1, "error in (no error)"=w427, "VISA resource name"=w426) -> ("error out"=w419:errorcluster)  [unwired: 6 in, 1 out]
                  }
                }
              }
            }
            "ob_temp" <- w391
            "cal_adc_delay" <- w388
          }
          frame #6 {
            # "if RX_FILT = -1 then use"
            # "freq driven filter select"
            n177 = local read "RX_FILT"() -> (w481:i32)
            n178 = case shown="-1" w481 {
              selector: w481 -> [w484 _]
              tunnel: [w485 w490] -> w482
              frame 0, Default {
                n179 = local write "RX_FILT"(w484) -> ()
                n180 = local read "RX_FILT(t)"() -> (w485:bool)
              }
              frame -1 {
                n181 = local read "Cutoff Freq (GHz)"() -> (w486:dbl)
                n182 = local read "RF_FREQ"() -> (w487:dbl)
                n183 = Greater Or Equal?(x=w487, y=w486) -> (x >= y?=w489:bool)
                n184 = call "Is Value Changed.vim"("value"=w489) -> ("changed or first call?"=w490:bool)
                n185 = case shown="False" w489 {
                  tunnel: [2 3] -> w488
                  frame False {
                  }
                  frame True {
                  }
                }
                n186 = local write "RX_FILT"(w488) -> ()
              }
            }
            "freq/filt change" <- w482
          }
          frame #7 {
            # "TEMP\nPS1-1_V\nRX_PORT\nREF_POWER\nRF_POWER\nRX_FILT\nRX_GAIN\nRF_FREQ"
            # "Make the path and filename for trace capture"
            n187 = local read "GET_TRACE"() -> (w495:bool)
            n188 = case shown="True" w495 {
              tunnel: [w496 w501] -> w494
              tunnel: w493 -> [w496 w498]
              frame False {
              }
              frame True {
                n189 = local read "Parameters"() -> (w508:string[])
                n190 = global read "Test Result File Name Global.vi" "Test Results File Name"() -> (w512:path)
                n191 = for {
                  tunnel: w508 -> [w527] mode=indexing
                  tunnel: [w525] -> w507 mode=indexing
                  n192 = Concatenate Strings(w527) -> (w526:string)
                  n193 = Search and Replace String(input string=w526, search string=".", replace string="p" ("replace string (\"\")")) -> (result string=w525:string)  [unwired: 5 in, 3 out]
                }
                n194 = Strip Path(path=w512) -> (stripped path=w513:path, name=w516:string)
                n195 = Search and Replace String(input string=w516, search string=".csv", replace string="_RxCaptureFiles" ("name or relative path"), error in=w498) -> (result string=w515:string, error out=w499:errorcluster)  [unwired: 4 in, 2 out]
                n196 = Build Path(base path=w513, name or relative path=w515) -> (appended path=w514:path)
                n197 = Array To Spreadsheet String(delimiter (Tab)="_", array=w507, 3:"%s" ("format string")) -> (spreadsheet string=w509:string)
                n198 = call <vilib>:"Check if File or Folder Exists.vi"("error in (no error)"=w499, "path"=w514) -> ("error out"=w500:errorcluster, "file or folder exists?"=w511:bool)  [unwired: 7 in, 1 out]
                n199 = case shown="True" w511 {
                  tunnel: w514 -> [w522 w524]
                  tunnel: [w521 w524] -> w517
                  tunnel: [w520 w523] -> w501
                  tunnel: w500 -> [w519 w523]
                  frame False {
                    n200 = Create Folder(path (use dialog)=w522, error in=w519) -> (created path=w521:path, error out=w520:errorcluster)  [unwired: 1 in, 1 out]
                  }
                  frame True {
                  }
                }
                n201 = call <vilib>:"Trim Whitespace.vi"("string"=w509) -> ("trimmed string"=w510:string)  [unwired: 1 in]
                n202 = Concatenate Strings(w510, ".csv" ("string")) -> (w518:string)
                n203 = Build Path(base path=w517, name or relative path=w518) -> (appended path=w497:path)
                "TraceFilePath" <- w497
                n204 = global write "Tetra_Globals.vi" "TraceFilePath"(w497) -> ()
              }
            }
          }
          frame #8 {
            # "Set the Power Supply"
            n205 = local read "V_SUPPLY(t)"() -> (w534:bool)
            n206 = local read "RF_FREQ"() -> (w533:dbl)
            n207 = First Call?() -> (First Call?: T/F=w531:bool)
            n208 = local write "RF_FREQ"(w533) -> ()
            n209 = Or(x=w531, y=w534) -> (x .or. y?=w530:bool)
            n210 = case shown="True" w530 {
              tunnel: [w536 w538] -> w535
              tunnel: w532 -> [w536 w537]
              frame False {
              }
              frame True {
                w541 = "PS1"  # SEL_PS
                n211 = local read "V_SUPPLY"() -> (w540:dbl)
                n212 = global read "Station References Global.vi" "PS1"() -> (w542:refnum<visa-resource-name>)
                n213 = call "INST_PS_SET_VOLTAGE_LEVEL_4.0.0.vi"("Instrument Select (Output 1)"="1", "SEL_PS"=w541, "error in (no error)"=w537, "Voltage (0.0)"=w540, "VISA session"=w542) -> ("error out"=w538:errorcluster)  [unwired: 5 in, 1 out]
              }
            }
          }
          frame #9 {
            n214 = local read "MODE"() -> (w543:bool)
            n215 = case shown="True" w543 {
              tunnel: [w546 w552] -> w545
              tunnel: w544 -> [w546 w551]
              frame False {
              }
              frame True {
                w548 = u16 1 items=["MHz", "GHz"] ("Freq Units")
                n216 = local read "comport"() -> (w550:refnum<visa-resource-name>)
                n217 = local read "RF_FREQ"() -> (w549:dbl)
                n218 = call "Tetra_Set-Freq.vi"("COMPORT"=w550, "error in (no error)"=w551, "Freq"=w549, "delay after set(ms)"=u32 10, "Freq Units"=w548) -> ("error out"=w552:errorcluster)  [unwired: 11 in, 3 out]
              }
            }
          }
          frame #10 {
            # "Set the PNA Stimulus"
            n219 = local read "RF_POWER(t)"() -> (w562:bool)
            n220 = case shown="True" w562 {
              tunnel: w564 -> [w592 w594]
              tunnel: [w592 w593] -> w563
              frame False {
              }
              frame True {
                # "Set the RF pow"
                n221 = global read "Station References Global.vi" "SigGen1"() -> (w596:refnum<visa-resource-name>)
                n222 = local read "RF_POWER"() -> (w595:dbl)
                n223 = call "VSG_SET-GET_AMPL_3.00.vi"("error in"=w594, "Set Power (num)"=w595, "Session In"=w596) -> ("error out"=w593:errorcluster)  [unwired: 6 in, 2 out]
              }
            }
            n224 = local read "RF_FREQ(t)"() -> (w565:bool)
            n225 = case shown="True" w565 {
              tunnel: w563 -> [w597 w601]
              tunnel: [w597 w599] -> w558
              frame False {
              }
              frame True {
                # "Set the RF Freq"
                n226 = global read "Station References Global.vi" "SigGen1"() -> (w602:refnum<visa-resource-name>)
                n227 = local read "RF_FREQ"() -> (w600:dbl)
                n228 = call "VSG_SET-GET_CW_1.00.vi"("Freq Units"="GHz", "error in"=w601, "Set Freq (MHz) num"=w600, "Session In"=w602) -> ("error out"=w599:errorcluster)  [unwired: 4 in, 3 out]
              }
            }
            n229 = local read "REF_PWR(t)"() -> (w561:bool)
            n230 = case shown="True" w561 {
              tunnel: w558 -> [w572 w573]
              tunnel: [w572 w576] -> w560
              frame False {
              }
              frame True {
                # "Set the ref pow"
                n231 = global read "Station References Global.vi" "PNA"() -> (w575:refnum<visa-resource-name>)
                n232 = local read "REF_POW"() -> (w579:dbl)
                n233 = call "Select Measurement.vi"("error in (no error)"=w573, "Measurement Name (CH1_S11_1)"="CH1_S11_1", "VISA resource name"=w575) -> ("error out"=w577:errorcluster, "VISA resource name out"=w574:refnum<visa-resource-name>)  [unwired: 7 in]
                n234 = call "Configure Power.vi"("VISA resource name"=w574, "error in (no error)"=w577, "Power Level (0 dBm)"=w579) -> ("error out"=w576:errorcluster)  [unwired: 11 in, 1 out]
              }
            }
            n235 = local read "ref_freq(t)"() -> (w559:bool)
            n236 = case shown="True" w559 {
              tunnel: w560 -> [w580 w585]
              tunnel: [w580 w590] -> w557
              frame False {
              }
              frame True {
                w581 = 1 ("Source")
                w583 = 0 items=["Normal", "SMC"] ("MODE")
                w589 = i64 1000000000 items=["GHz"=1000000000, "MHZ"=1000000] ("Units")
                # "Set the ref Freq"
                n237 = global read "Station References Global.vi" "PNA"() -> (w586:refnum<visa-resource-name>)
                n238 = local read "ref_freq"() -> (w591:dbl)
                n239 = call "Select Measurement.vi"("error in (no error)"=w585, "Measurement Name (CH1_S11_1)"="CH1_S11_1", "Channel (1)"=1, "VISA resource name"=w586) -> ("error out"=w588:errorcluster, "VISA resource name out"=w587:refnum<visa-resource-name>)  [unwired: 6 in]
                n240 = call "PNA-L_SET-CWFREQ.vi"("Session In"=w587, "error in"=w588, "MODE"=w583, "FREQ"=w591, "Units"=w589, "CH"=w581, "Source"=w581) -> ("error out"=w590:errorcluster)  [unwired: 10 in, 2 out]
              }
            }
            n241 = local read "REF_PWR(t)"() -> (w555:bool)
            n242 = local read "ref_freq(t)"() -> (w554:bool)
            n243 = Or(x=w555, y=w554) -> (x .or. y?=w553:bool)
            n244 = case shown="True" w553 {
              tunnel: w557 -> [w566 w570]
              tunnel: [w566 w569] -> w556
              frame False {
              }
              frame True {
                w567 = 3 items=["HOLD", "CONT", "GROUP", "SINGLE"] ("Mode")
                # "take a sweep to make the changes"
                n245 = global read "Station References Global.vi" "PNA"() -> (w571:refnum<visa-resource-name>)
                n246 = call "PNA_SWEEP MODE.vi"("Mode"=w567, "Channel"=1 ("Source"), "error in (no error)"=w570, "VISA resource name"=w571) -> ("error out"=w569:errorcluster)  [unwired: 6 in, 1 out]
              }
            }
          }
          frame #11 {
            # "Set ADAR values"
            n247 = local read "RX_PORT(t)"() -> (w609:bool)
            n248 = case shown="True" w609 {
              tunnel: w615 -> [w685 w689]
              tunnel: [w685 w688] -> w613
              frame False {
              }
              frame True {
                w692 = 0 items=["RX", "TX"] ("RX/TX")
                n249 = local read "RX_PORT"() -> (w691:i32)
                n250 = local read "comport"() -> (w690:refnum<visa-resource-name>)
                n251 = global read "Tetra_Globals.vi" "RevC(t)"() -> (w686:bool)
                n252 = call "Tetra_AntSel.vi"("COMPORT"=w690, "REVC(T)"=w686, "error in (no error)"=w689, "RX/TX"=w692, "ANT(num)"=w691, "milliseconds to wait"=u32 10) -> ("error out"=w688:errorcluster)  [unwired: 11 in, 2 out]
              }
            }
            n253 = local read "freq/filt change"() -> (w612:bool)
            n254 = local read "MODE"() -> (w606:bool)
            n255 = case shown="True" w606 {
              tunnel: w613 -> [w620 w646]
              tunnel: w612 -> [w619 _]
              tunnel: [w618 w641] -> w611
              tunnel: [w617 w645] -> w607
              tunnel: [-1 ("bpf") w636] -> w605
              frame False {
                n256 = case shown="True" w619 {
                  tunnel: w620 -> [w622 w631]
                  tunnel: [w622 w630] -> w618
                  tunnel: [w621 w626] -> w617
                  frame False {
                    n257 = local read "RX_FILT"() -> (w621:i32)
                  }
                  frame True {
                    w628 = 0 items=["RX", "TX"] ("RX/TX")
                    n258 = local read "RX_PORT"() -> (w623:i32)
                    n259 = local read "comport"() -> (w629:refnum<visa-resource-name>)
                    n260 = global read "Tetra_Globals.vi" "RevC(t)"() -> (w624:bool)
                    n261 = local read "RX_FILT"() -> (w625:i32)
                    n262 = call "Tx-RxFilt.vi"("COMPORT"=w629, "REVC(T)"=w624, "AntPort"=w623, "error in (no error)"=w631, "RX/TX"=w628, "VERIFY(t)"=TRUE, "Filt(sel)"=w625) -> ("filt(num)"=w626:i32, "error out"=w630:errorcluster)  [unwired: 10 in, 1 out]
                  }
                }
              }
              frame True {
                w635 = u32 10 ("milliseconds to wait")
                w638 = 0 items=["RX", "TX"] ("RX/TX")
                w643 = 0 items=["RX", "TX"] ("RX/TX")
                n263 = local read "comport"() -> (w644:refnum<visa-resource-name>)
                n264 = global read "Tetra_Globals.vi" "RevC(t)"() -> (w634:bool)
                n265 = local read "RX_PORT"() -> (w633:i32)
                n266 = call "Tx-RxFilt.vi"("COMPORT"=w644, "REVC(T)"=w634, "AntPort"=w633, "error in (no error)"=w646, "RO(t)"=TRUE ("VERIFY(t)"), "RX/TX"=w643, "VERIFY(t)"=FALSE, "milliseconds to wait"=w635) -> ("filt(num)"=w645:i32, "comport"=w639:refnum<visa-resource-name>, "error out"=w640:errorcluster)  [unwired: 9 in]
                n267 = call "Tetra_BPF.vi"("COMPORT"=w639, "Rev-C(t)"=w634, "ant-port"=w633, "error in (no error)"=w640, "RO(t)"=TRUE, "RX/TX"=w638, "milliseconds to wait"=w635) -> ("bpf"=w636:i32, "error out"=w641:errorcluster)  [unwired: 10 in, 1 out]
              }
            }
            "rx_filt" <- w607
            "bpf" <- w605
            n268 = local read "rx_gain_auto(t)"() -> (w603:bool)
            n269 = local read "MODE"() -> (w608:bool)
            n270 = And(x=w608, y=w603) -> (x .and. y?=w604:bool)
            n271 = case shown="True" w604 {
              tunnel: w611 -> [w655 w683]
              tunnel: [w654 w684] -> w614
              tunnel: [w652 w680] -> w610
              tunnel: w603 -> [w648 _]
              frame False {
                n272 = local read "RX_PORT(t)"() -> (w650:bool)
                n273 = local read "RX_GAIN(t)"() -> (w651:bool)
                n274 = Or(x=w650, y=w651) -> (x .or. y?=w653:bool)
                n275 = Not(x=w648) -> (.not. x?=w647:bool)
                n276 = Or(x=w653, y=w647) -> (x .or. y?=w649:bool)
                n277 = case shown="True" w649 {
                  tunnel: w655 -> [w657 w663]
                  tunnel: [w657 w662] -> w654
                  tunnel: [i32[] [-1, -1, -1, -1] ("Readback (1-4)") w660] -> w652
                  frame False {
                  }
                  frame True {
                    n278 = local read "RX_PORT"() -> (w661:i32)
                    n279 = local read "RX_GAIN"() -> (w659:i32)
                    n280 = global read "Tetra_Globals.vi" "RevC(t)"() -> (w658:bool)
                    n281 = case shown="0.." w659 {
                      tunnel: w659 -> [w670 w677]
                      tunnel: w663 -> [w669 w676]
                      tunnel: [w668 w675] -> w662
                      tunnel: w661 -> [w667 w674]
                      tunnel: [w666 w673] -> w660
                      tunnel: w658 -> [w664 w672]
                      frame -1, Default {
                        n282 = local read "comport"() -> (w671:refnum<visa-resource-name>)
                        n283 = call "Tetra_RxGain.vi"("COMPORT"=w671, "error in (no error)"=w669, "RXPORT(num)"=w667, "GAIN(code)"=w670, "REVC(T)"=w664, "RO(t)"=TRUE) -> ("Readback (1-4)"=w666:i32[], "error out"=w668:errorcluster)  [unwired: 9 in, 3 out]
                      }
                      frame 0.. {
                        n284 = local read "comport"() -> (w678:refnum<visa-resource-name>)
                        n285 = call "Tetra_RxGain.vi"("COMPORT"=w678, "error in (no error)"=w676, "RXPORT(num)"=w674, "GAIN(code)"=w677, "REVC(T)"=w672) -> ("Readback (1-4)"=w673:i32[], "error out"=w675:errorcluster)  [unwired: 10 in, 3 out]
                      }
                    }
                  }
                }
              }
              frame True {
                n286 = local read "comport"() -> (w682:refnum<visa-resource-name>)
                n287 = global read "Tetra_Globals.vi" "RevC(t)"() -> (w679:bool)
                n288 = call "Tetra_RxGain.vi"("COMPORT"=w682, "error in (no error)"=w683, "REVC(T)"=w679, "RO(t)"=TRUE) -> ("Readback (1-4)"=w680:i32[], "error out"=w684:errorcluster)  [unwired: 11 in, 3 out]
              }
            }
            "rxgain (1-4)" <- w610
          }
          frame #12 {
            n289 = local read "MEAS_PS"() -> (w702:bool)
            n290 = local read "V_SUPPLY(t)"() -> (w703:bool)
            n291 = First Call?() -> (First Call?: T/F=w695:bool)
            n292 = Or(x=w695, y=w702) -> (x .or. y?=w696:bool)
            n293 = local read "RX_PORT(t)"() -> (w693:bool)
            n294 = Or(x=w696, y=w703) -> (x .or. y?=w701:bool)
            n295 = Or(x=w701, y=w693) -> (x .or. y?=w694:bool)
            n296 = case shown="True" w694 {
              tunnel: [-1.0 w710] -> w698
              tunnel: [w708 w711] -> w705
              tunnel: w704 -> [w708 w712]
              tunnel: [1.0 ("V_SUPPLY") w709] -> w700
              frame False {
              }
              frame True {
                w713 = TRUE  # Clear Error in
                w714 = 0.05  # Delay Time (s)
                w718 = 0 items=["Current", "Voltage"] ("Measurement Type (1: Voltage)")
                w719 = "PS1"  # SEL_PS
                n297 = call "Time Delay2"("error in (no error)"=w712, "Delay Time (s)"=w714) -> ("error out"=w715:errorcluster)  [unwired: 9 in]
                n298 = global read "Station References Global.vi" "PS1"() -> (w716:refnum<visa-resource-name>)
                n299 = local read "V_SUPPLY"() -> (w709:dbl)
                n300 = call "INST_PS_MEAS_3.0.0.vi"("VISA session"=w716, "Clear Error in"=w713, "SEL_PS"=w719, "Channel Name (1)"="1", "error in (no error)"=w715, "Measurement Type (1: Voltage)"=w718) -> ("Measurement"=w710:dbl, "error out"=w711:errorcluster)  [unwired: 6 in, 2 out]
              }
            }
            n301 = Multiply(x=w698, y=w700) -> (x*y=w699:dbl)
            n302 = Build Array(w698, w699) -> (→"ps_meas(i)(w)":dbl[])
          }
          frame #13 {
            n303 = flat-sequence {
              tunnel: w726 -> [w735]
              tunnel: [w739] -> w725
              tunnel: [w729] -> w724
              tunnel: w725 -> [w806]
              tunnel: w724 -> [w801]
              tunnel: [w803] -> w723
              tunnel: w723 -> [w860]
              tunnel: [w861] -> w722
              tunnel: w722 -> [w868]
              tunnel: [w869] -> w720
              tunnel: [w946] -> w721
              tunnel: w720 -> [w946]
              frame #0 {
                # "Get the RX Data"
                # "Get Signal Power"
                n304 = case shown="True" TRUE {
                  tunnel: w735 -> [w746 w750]
                  tunnel: [w746 w756] -> w739
                  tunnel: [w744 w751] -> w742
                  tunnel: [w744 w757] -> w741
                  tunnel: [w744 w752] -> w740
                  tunnel: [w744 w754] -> w736
                  tunnel: [w743 w749] -> w732
                  tunnel: ["-1" ("chan_id") w755] -> w738
                  tunnel: [w743 w753] -> w734
                  tunnel: [w743 w748] -> w731
                  frame False {
                    w743 = FALSE ("unlocked(t)")
                    w744 = -1.0 ("rx_span")
                  }
                  frame True {
                    n305 = for {
                      N: 1 -> [_]
                      tunnel: [w800] -> w757
                      tunnel: [w794] -> w755
                      tunnel: [w793] -> w754
                      tunnel: [w790] -> w753
                      tunnel: [w775] -> w752
                      tunnel: [w774] -> w751
                      tunnel: [w764] -> w749
                      tunnel: [w763] -> w748
                      shift-right: [w797] -> w756
                      shift-left: w750 -> [w767]
                      i -> [w759]
                      stop <- w763 stop-if-true
                      w782 = ".csv" ("search string")
                      # "IF adc_lock = T\nAND f_lock = T\nTHEN = F"
                      n306 = local read "TraceFilePath"() -> (w789:path)
                      n307 = global read "Sequence Globals.vi" "Current Iteration"() -> (w776:i32)
                      n308 = Greater Than 0?(x=w759) -> (x > 0?=w760:bool)
                      n309 = disable-structure shown="Enabled" {
                        frame Disabled {
                          n310 = local read "RunAM_Init"() -> ()  [unwired: 1 out]
                        }
                        frame Enabled {
                        }
                      }
                      n311 = Path To String(path=w789) -> (string=w784:string)
                      n312 = local read "RunAM_Init"() -> (w762:bool)
                      n313 = Empty String/Path?(string/path=w784) -> (empty?=w773:bool)
                      n314 = Search and Replace String(input string=w784, search string=w782) -> (result string=w787:string)  [unwired: 6 in, 3 out]
                      n315 = Format Into String(initial string="_", w776) -> (resulting string=w781:string)  [unwired: 2 in, 1 out]
                      n316 = Or(x=w760, y=w762) -> (x .or. y?=w761:bool)
                      n317 = Equal To 0?(x=w759) -> (x = 0?=w758:bool)
                      n318 = local read "RX_PORT"() -> (w765:i32)
                      n319 = Concatenate Strings(w787, "_sigcapt" ("string"), w781, w782) -> (w771:string)
                      n320 = Select(t="-1", s=w773, f=w771) -> (s? t:f=w770:string)
                      "sigcapture path" <- w770
                      n321 = local read "ADC_ETH(T)"() -> (w778:bool)
                      n322 = local read "GET_TRACE"() -> (w779:bool)
                      n323 = local read "BW(MHz)"() -> (w798:dbl)
                      n324 = local read "dBFS_REF"() -> (w777:dbl)
                      n325 = String To Path(string=w770) -> (path=w780:path)
                      n326 = local read "if_freq"() -> (w799:dbl)
                      n327 = local read "#OFAVGs-Sig"() -> (w769:i32)
                      n328 = local read "MEAS_SNR"() -> (w795:bool)
                      n329 = local read "comport"() -> (w792:refnum<visa-resource-name>)
                      n330 = global read "Tetra_Globals.vi" "RevC(t)"() -> (w766:bool)
                      n331 = call "GetRxPower(LC).vi"("SAVE FILE PATH"=w780, "CloseCOM4"=w758, "RXAnt"=w765, "RunAM_Init"=w761, "UseFastData(T)"=w778, "error in (no error)"=w767, "dBFS Ofset"=w777, "SAVE TO FILE(T)"=w779, "CF(MHZ)"=w799, "BW(MHZ)"=w798, "#ofAvg"=w769) -> ("band (dbfs/mhz)"=w785:dbl[], "peak (dbfs/mhz)"=w786:dbl[], "Locked?(T)"=w764:bool, "Am_Init_Flag"=w768:bool, "error out"=w796:errorcluster)  [unwired: 4 in]
                      n332 = Index Array(array=w785) -> (element #1=w774:dbl, element #2=w800:dbl)  [unwired: 2 in]
                      n333 = Index Array(array=w786) -> (element #1=w775:dbl, element #2=w793:dbl)  [unwired: 2 in]
                      n334 = local write "RunAM_Init"(w768) -> ()
                      n335 = call "Tetra_ADC-Frame.vi"("COMPORT"=w792, "error in (no error)"=w796, "Execute"=w766, "Open Ser(t)"=TRUE ("RunAM_Init"), "Close Ser(t)"=w795) -> ("locked(t)"=w790:bool, "chan_id"=w794:string, "error out"=w797:errorcluster)  [unwired: 7 in, 1 out]
                      n336 = And(x=w790, y=w764) -> (x .and. y?=w763:bool)
                    }
                  }
                }
                "rxpeak_dbm" <- w740
                "rxpeak_mhz" <- w736
                "rx_bpower_on" <- w742
                "fout_bp" <- w741
                "adc_lock(t)" <- w734
                "adc_chan_id" <- w738
                "freq_lock(t)" <- w732
                n337 = local read "ADC_SYNC_NOT"() -> (w737:bool)
                n338 = global read "Tetra_Globals.vi" "RevC(t)"() -> (w728:bool)
                n339 = Or(x=w731, y=w737) -> (x .or. y?=w730:bool)
                n340 = Select(t=w730, s=w728, f=TRUE) -> (s? t:f=w729:bool)
              }
              frame #1 {
                # "force to TRUE to skip the retry"
                # "IF ADC did not sync"
                # "ADC SYNC NOT USED"
                n341 = case shown="False" w801 {
                  tunnel: w806 -> [w814 w859]
                  tunnel: [w820 w859] -> w803
                  tunnel: [w815 "-1" ("output")] -> w804
                  tunnel: [w807 -1] -> w805
                  frame False {
                    n342 = local read "BW(MHz)"() -> (w823:dbl)
                    n343 = local read "#of_adc-resyncs"() -> (w808:i32)
                    n344 = local read "if_freq"() -> (w824:dbl)
                    n345 = for {
                      N: w808 -> [w846]
                      tunnel: [w836] -> w819
                      tunnel: [w856] -> w816
                      shift-right: [w839] -> w821
                      shift-left: w814 -> [w848]
                      tunnel: [w835] -> w817
                      tunnel: [w853] -> w818
                      tunnel: w824 -> [w852]
                      tunnel: w823 -> [w851]
                      tunnel: [w849] -> w815
                      tunnel: [w829] -> w807
                      i -> [w843]
                      stop <- w847 stop-if-true
                      n346 = local read "ADC_ETH(T)"() -> (w830:bool)
                      n347 = local read "GET_TRACE"() -> (w842:bool)
                      n348 = local read "dBFS_REF"() -> (w837:dbl)
                      n349 = local read "sigcapture path"() -> (w841:string)
                      n350 = local read "RX_PORT"() -> (w831:i32)
                      n351 = local read "comport"() -> (w850:refnum<visa-resource-name>)
                      n352 = String To Path(string=w841) -> (path=w840:path)
                      n353 = call "ADCSync_LC.vi"("COMPORT"=w850, "ClearErrorIn(t)"=TRUE, "error in (no error)"=w848, "revc(t)"=TRUE, "Open Ser(t)"=TRUE, "Close Ser(t)"=FALSE) -> ("output"=w849:string, "error out"=w832:errorcluster)  [unwired: 5 in, 3 out]
                      n354 = Increment(x=w843) -> (x+1=w829:i32)
                      n355 = Equal?(x=w829, y=w846) -> (x = y?=w845:bool)
                      n356 = call "GetRxPower(LC).vi"("SAVE FILE PATH"=w840, "CloseCOM4"=FALSE, "RXAnt"=w831, "RunAM_Init"=TRUE, "UseFastData(T)"=w830, "error in (no error)"=w832, "dBFS Ofset"=w837, "SAVE TO FILE(T)"=w842, "CF(MHZ)"=w852, "BW(MHZ)"=w851, "#ofAvg"=1) -> ("band (dbfs/mhz)"=w854:dbl[], "peak (dbfs/mhz)"=w855:dbl[], "Locked?(T)"=w844:bool, "error out"=w839:errorcluster)  [unwired: 4 in, 1 out]
                      n357 = Or(x=w844, y=w845) -> (x .or. y?=w847:bool)
                      n358 = Index Array(array=w855) -> (element #1=w836:dbl, element #2=w856:dbl)  [unwired: 2 in]
                      n359 = Index Array(array=w854) -> (element #1=w835:dbl, element #2=w853:dbl)  [unwired: 2 in]
                    }
                    n360 = local read "MEAS_SNR"() -> (w810:bool)
                    n361 = local read "comport"() -> (w813:refnum<visa-resource-name>)
                    n362 = global read "Tetra_Globals.vi" "RevC(t)"() -> (w809:bool)
                    n363 = local write "rx_bpower_on"(w817) -> ()
                    n364 = local write "fout_bp"(w818) -> ()
                    n365 = local write "rxpeak_dbm"(w819) -> ()
                    n366 = local write "rxpeak_mhz"(w816) -> ()
                    n367 = call "Tetra_ADC-Frame.vi"("COMPORT"=w813, "error in (no error)"=w821, "Execute"=w809, "Open Ser(t)"=TRUE, "Close Ser(t)"=w810) -> ("locked(t)"=w811:bool, "chan_id"=w812:string, "error out"=w820:errorcluster)  [unwired: 7 in, 1 out]
                    n368 = local write "adc_lock(t)"(w811) -> ()
                    n369 = local write "adc_chan_id"(w812) -> ()
                  }
                  frame True {
                  }
                }
                "adc#ofresync" <- w805
                n370 = call <vilib>:"Trim Whitespace.vi"("string"=w804) -> ("trimmed string"=→"adcsync":string)  [unwired: 1 in]
              }
              frame #2 {
                n371 = flat-sequence {
                  tunnel: w860 -> [w863]
                  tunnel: [w863] -> w861
                  frame #0 {
                    # "Compute Gain"
                    n372 = local read "rxpeak_dbm"() -> (w865:dbl)
                    n373 = local read "RF_POWER"() -> (w864:dbl)
                    n374 = Subtract(x=w865, y=w864) -> (x-y=→"peak_gain":dbl)
                  }
                }
              }
              frame #3 {
                # "MEASURE NOISE FIGURE"
                n375 = local read "MEAS_SNR"() -> (w867:bool)
                n376 = case shown="True" w867 {
                  tunnel: [w874 w881] -> w869
                  tunnel: [w875 w880] -> w870
                  tunnel: [w875 w882] -> w871
                  tunnel: w868 -> [w874 w898]
                  tunnel: [FALSE ("Am_Init_Flag") w879] -> w866
                  frame False {
                    w875 = -1.0 ("rx_span")
                    n377 = local write "noisecapture path"("-1" ("noisecapture path")) -> ()
                  }
                  frame True {
                    w890 = ".csv" ("search string")
                    n378 = global read "Station References Global.vi" "SigGen1"() -> (w900:refnum<visa-resource-name>)
                    n379 = call "VSG_SET_RF_STATE_1.00.vi"("RF ON/OFF (OFF)"=FALSE, "error in"=w898, "Session In"=w900) -> ("error out"=w878:errorcluster)  [unwired: 6 in, 2 out]
                    n380 = flat-sequence {
                      tunnel: w878 -> [w916]
                      tunnel: [w905] -> w877
                      tunnel: [w928] -> w885
                      tunnel: [w921] -> w883
                      tunnel: [w921] -> w880
                      tunnel: [w920] -> w879
                      tunnel: w877 -> [w929]
                      tunnel: w876 -> [w919]
                      tunnel: w885 -> [w935]
                      tunnel: [w935] -> w884
                      tunnel: w883 -> [w932]
                      tunnel: [w934] -> w882
                      tunnel: w884 -> [w939]
                      tunnel: [w937] -> w886
                      tunnel: w886 -> [w943]
                      tunnel: [w941] -> w881
                      frame #0 {
                        w901 = 3 items=["HOLD", "CONT", "GROUP", "SINGLE"] ("Mode")
                        w902 = 1 ("Source")
                        w910 = 0 items=["Normal", "SMC"] ("MODE")
                        w915 = i64 1000000000 items=["GHz"=1000000000, "MHZ"=1000000] ("Units")
                        # "Set the ref Freq"
                        n381 = local read "NF_OFS_GHZ"() -> (w906:dbl)
                        n382 = local read "ref_freq"() -> (w908:dbl)
                        n383 = global read "Station References Global.vi" "PNA"() -> (w912:refnum<visa-resource-name>)
                        n384 = Subtract(x=w908, y=w906) -> (x-y=w907:dbl)
                        n385 = call "Select Measurement.vi"("error in (no error)"=w916, "Measurement Name (CH1_S11_1)"="CH1_S11_1", "Channel (1)"=1, "VISA resource name"=w912) -> ("error out"=w914:errorcluster, "VISA resource name out"=w913:refnum<visa-resource-name>)  [unwired: 6 in]
                        n386 = call "PNA-L_SET-CWFREQ.vi"("Session In"=w913, "error in"=w914, "MODE"=w910, "FREQ"=w907, "Units"=w915, "CH"=w902, "Source"=w902) -> ("Session Out"=w903:refnum<visa-resource-name>, "error out"=w904:errorcluster)  [unwired: 10 in, 1 out]
                        n387 = call "PNA_SWEEP MODE.vi"("Mode"=w901, "Channel"=w902, "error in (no error)"=w904, "VISA resource name"=w903) -> ("error out"=w905:errorcluster)  [unwired: 6 in, 1 out]
                      }
                      frame #1 {
                        n388 = local read "ADC_ETH(T)"() -> (w924:bool)
                        n389 = local read "GET_TRACE"() -> (w927:bool)
                        n390 = local read "BW(MHz)"() -> (w930:dbl)
                        n391 = local read "dBFS_REF"() -> (w923:dbl)
                        n392 = String To Path(string=w919) -> (path=w926:path)
                        n393 = local read "RX_PORT"() -> (w918:i32)
                        n394 = local read "if_freq"() -> (w931:dbl)
                        n395 = local read "#OFAVGs-Noi"() -> (w922:i32)
                        n396 = call "GetRxPower(LC).vi"("SAVE FILE PATH"=w926, "RXAnt"=w918, "RunAM_Init"=TRUE, "UseFastData(T)"=w924, "error in (no error)"=w929, "dBFS Ofset"=w923, "SAVE TO FILE(T)"=w927, "CF(MHZ)"=w931, "BW(MHZ)"=w930, "#ofAvg"=w922) -> ("band (dbfs/mhz)"=w925:dbl[], "Am_Init_Flag"=w920:bool, "error out"=w928:errorcluster)  [unwired: 5 in, 2 out]
                        n397 = Index Array(array=w925) -> (element #1=w921:dbl)  [unwired: 2 in, 1 out]
                      }
                      frame #2 {
                        n398 = local read "rx_bpower_on"() -> (w933:dbl)
                        n399 = Subtract(x=w933, y=w932) -> (x-y=w934:dbl)
                      }
                      frame #3 {
                        n400 = global read "Station References Global.vi" "SigGen1"() -> (w938:refnum<visa-resource-name>)
                        n401 = call "VSG_SET_RF_STATE_1.00.vi"("RF ON/OFF (OFF)"=TRUE, "error in"=w939, "Session In"=w938) -> ("error out"=w937:errorcluster)  [unwired: 6 in, 2 out]
                      }
                      frame #4 {
                        n402 = local read "comport"() -> (w940:refnum<visa-resource-name>)
                        n403 = call "Tetra Serial.vi"("COMPORT"=w940, "error in (no error)"=w943, "Open Ser(t)"=TRUE) -> ("error out"=w941:errorcluster)  [unwired: 8 in, 4 out]
                      }
                    }
                    n404 = local read "TraceFilePath"() -> (w897:path)
                    n405 = global read "Sequence Globals.vi" "Current Iteration"() -> (w892:i32)
                    n406 = Path To String(path=w897) -> (string=w894:string)
                    n407 = Empty String/Path?(string/path=w894) -> (empty?=w893:bool)
                    n408 = Search and Replace String(input string=w894, search string=w890) -> (result string=w895:string)  [unwired: 6 in, 3 out]
                    n409 = Format Into String(initial string="_", w892) -> (resulting string=w889:string)  [unwired: 2 in, 1 out]
                    n410 = Concatenate Strings(w895, "_noisecapt" ("string"), w889, w890) -> (w887:string)
                    n411 = Select(t="-1", s=w893, f=w887) -> (s? t:f=w876:string)
                    "noisecapture path" <- w876
                  }
                }
                "rx_bpower_off" <- w870
                "s-n" <- w871
                n412 = local write "RunAM_Init"(w866) -> ()
              }
              frame #4 {
                n413 = local read "MEAS_SNR"() -> (w944:bool)
                n414 = case shown="False" w944 {
                  tunnel: [-1.0 w949] -> w945
                  frame False {
                  }
                  frame True {
                    n415 = local read "rx_bpower_off"() -> (w950:dbl)
                    n416 = local read "peak_gain"() -> (w951:dbl)
                    n417 = local read "BW(MHz)"() -> (w948:dbl)
                    n418 = call "NF_CALC.vi"("G(db)"=w951, "BW(MHz)"=w948, "BandPow(dBm)"=w950) -> ("NF(dB)"=w949:dbl)  [unwired: 8 in]
                  }
                }
                "nf" <- w945
              }
            }
          }
          frame #14 {
            n419 = local read "MEAS_ADAR_TEMP"() -> (w957:bool)
            n420 = local read "RX_PORT(t)"() -> (w952:bool)
            n421 = First Call?() -> (First Call?: T/F=w954:bool)
            n422 = Or(x=w954, y=w957) -> (x .or. y?=w955:bool)
            n423 = Or(x=w952, y=w955) -> (x .or. y?=w953:bool)
            n424 = case shown="True" w953 {
              tunnel: [w960 w964] -> w958
              tunnel: [dbl[] [-1.0, -1.0, -1.0, -1.0, -1.0, -1.0] w967] -> w956
              tunnel: w959 -> [w960 w973]
              frame False {
              }
              frame True {
                n425 = local read "RX_PORT"() -> (w963:i32)
                n426 = local read "comport"() -> (w974:refnum<visa-resource-name>)
                n427 = global read "Tetra_Globals.vi" "RevC(t)"() -> (w962:bool)
                n428 = call "RX-ADAR-TEMP.vi"("COMPORT"=w974, "RevC(t)"=w962, "error in (no error)"=w973, "RxPort"=w963) -> ("comport"=w971:refnum<visa-resource-name>, "temp(c)"=w968:dbl, "error out"=w970:errorcluster)  [unwired: 8 in, 1 out]
                n429 = call "ReadTempSense.vi"("COMPORT"=w971, "error in (no error)"=w970) -> ("temp(c)"=w969:dbl[], "error out"=w966:errorcluster)  [unwired: 10 in, 2 out]
                n430 = call "Time Delay3"("error in (no error)"=w966, "Delay Time (s)"=0.01) -> ("error out"=w964:errorcluster)  [unwired: 9 in]
                n431 = Insert Into Array(array=w969, index=0, new element=w968) -> (w967:dbl[])
              }
            }
            "temp_sense1-2" <- w956
          }
          frame #15 {
            n432 = local read "MEAS_DCMON"() -> (w977:bool)
            n433 = local read "V_SUPPLY(t)"() -> (w978:bool)
            n434 = local read "RX_PORT(t)"() -> (w975:bool)
            n435 = Or(x=w977, y=w978) -> (x .or. y?=w979:bool)
            n436 = Or(x=w979, y=w975) -> (x .or. y?=w976:bool)
            n437 = case shown="True" w976 {
              tunnel: [w991 w1006] -> w984
              tunnel: [w991 w1005] -> w983
              tunnel: [w989 w1004] -> w982
              tunnel: [w992 w1002] -> w981
              tunnel: w980 -> [w989 w997]
              frame False {
                n438 = global read "Tetra_Globals.vi" "RevC(t)"() -> (w985:bool)
                n439 = Select(t=11, s=w985, f=11) -> (s? t:f=w988:i32)
                n440 = for {
                  N: 6 -> [_]
                  tunnel: [-1.0] -> w991 mode=indexing
                }
                n441 = for {
                  N: w988 -> [_]
                  tunnel: [-1.0] -> w992 mode=indexing
                }
              }
              frame True {
                n442 = local read "comport"() -> (w1003:refnum<visa-resource-name>)
                n443 = call "Tetra_Read UCD.vi"("COMPORT"=w1003, "error in (no error)"=w997) -> ("rdv"=w1002:dbl[], "comport"=w1000:refnum<visa-resource-name>, "error out"=w1001:errorcluster)  [unwired: 11 in]
                n444 = global read "Tetra_Globals.vi" "RevC(t)"() -> (w995:bool)
                n445 = call "Time Delay"("error in (no error)"=w1001, "Delay Time (s)"=0.01) -> ("error out"=w999:errorcluster)  [unwired: 9 in]
                n446 = call "Tetra_Read Imon.vi"("COMPORT"=w1000, "rev_c(t)"=w995, "error in (no error)"=w999, "Meas_Limits"=FALSE) -> ("rdiv(i)"=w1006:dbl[], "rdiv(v)"=w1005:dbl[], "error out"=w1004:errorcluster)  [unwired: 10 in, 3 out]
              }
            }
            "rdiv(i)" <- w984
            "rdiv(v)" <- w983
            "rdv" <- w981
          }
          frame #16 {
            n447 = flat-sequence {
              tunnel: [w1009] -> _
              tunnel: [w1009] -> w1007
              frame #0 {
                w1010 = TRUE ("Close Serial")
                # "Check the Safety System"
                n448 = local read "ess_error"() -> (w1015:errorcluster)
                n449 = global read "Station References Global.vi" "Gantry"() -> (w1013:refnum<visa-resource-name>)
                n450 = local read "FH_NOT(T)"() -> (w1012:bool)
                n451 = call "WAM_ESS.vi"("VISA resource name"=w1013, "error in (no error)"=w1015, "Open Serial"=w1010, "Test Running (T)"=w1010, "Close Serial"=w1010) -> ("FH_NOT(T)"=w1011:bool, "VISA resource name out"=w1014:refnum<visa-resource-name>, "error out"=w1016:errorcluster)  [unwired: 7 in, 1 out]
                n452 = And(x=w1012, y=w1011) -> (x .and. y?=w1009:bool)
                "no_fault" <- w1009
                n453 = case shown="True" w1009 {
                  tunnel: w1014 -> [w1025 _]
                  tunnel: w1016 -> [w1024 w1031]
                  tunnel: [w1023 w1031] -> w1017
                  frame False {
                    w1021 = u16 1 items=["Disable Driver", "Enable Driver", "Read Driver Status"] ("Driver-Func")
                    w1022 = TRUE ("Close Serial")
                    n454 = call "Prompt User for Input"("error in (no error)"=w1024) -> ("OK"=w1020:bool, "error out"=w1019:errorcluster)  [unwired: 17 in]
                    n455 = case shown="False" w1020 {
                      selector: w1020 -> [w1027 _]
                      tunnel: w1019 -> [w1029 w1030]
                      tunnel: [w1028 w1030] -> w1018
                      frame False {
                        n456 = invoke class="VI" method="Abort VI"(error in=w1029) -> (error out=w1028:errorcluster)  [unwired: 2 in, 2 out]
                        n457 = Not(x=w1027) -> (.not. x?=w1026:bool)
                        n458 = local write "STOP(T)"(w1026) -> ()
                        n459 = global write "Sequence Globals.vi" "Stop Testing"(w1026) -> ()
                      }
                      frame True {
                      }
                    }
                    n460 = call "Gantry_Driver.vi"("VISA resource name"=w1025, "error in (no error)"=w1018, "Open Serial"=w1022, "Driver-Func"=w1021, "Close Serial"=w1022) -> ("error out"=w1023:errorcluster)  [unwired: 11 in, 3 out]
                  }
                  frame True {
                  }
                }
                n461 = local write "ess_error"(w1017) -> ()
              }
            }
          }
          frame #17 {
            n462 = local read "ser_rd"() -> (w1033:string)
            n463 = Empty String/Path?(string/path=w1033) -> (empty?=w1034:bool)
            n464 = case shown="True" w1034 {
              tunnel: [w1037 "null" ("result string")] -> w1032
              tunnel: w1033 -> [w1043 _]
              frame False {
                w1036 = TRUE ("replace all? (F)")
                n465 = local read "comport"() -> (w1044:refnum<visa-resource-name>)
                n466 = call "SerRW-Array.vi"("COMPORT"=w1044, "Command ( ; seperation)"=w1043) -> ("string"=w1041:string)  [unwired: 7 in, 6 out]
                n467 = call <vilib>:"Space Constant.vi"() -> ("String"=w1038:string)
                n468 = Search and Replace String(replace all?=w1036, input string=w1041, search string="\n", replace string=w1038) -> (result string=w1040:string)  [unwired: 4 in, 3 out]
                n469 = Search and Replace String(replace all?=w1036, input string=w1040, search string="\r", replace string=w1038) -> (result string=w1037:string)  [unwired: 4 in, 3 out]
              }
              frame True {
              }
            }
            "readback" <- w1032
          }
          frame #18 {
            w1055 = T1 2 items=["both", "start of string", "end of string"] ("location (both)")
            n470 = local read "relative seconds"() -> (w1096:dbl)
            n471 = local read "freq_lock(t)"() -> (w1049:bool)
            n472 = global read "Sequence Globals.vi" "Current Iteration"() -> (w1095:i32)
            n473 = local read "temp_sense1-2"() -> (w1077:dbl[])
            n474 = local read "rx_bpower_on"() -> (w1088:dbl)
            n475 = local read "rx_bpower_off"() -> (w1086:dbl)
            n476 = local read "ps_meas(i)(w)"() -> (w1090:dbl[])
            n477 = call <vilib>:"High Resolution Relative Seconds.vi"() -> ("relative seconds"=w1097:dbl)
            n478 = local read "rxpeak_dbm"() -> (w1081:dbl)
            n479 = local read "rxpeak_mhz"() -> (w1080:dbl)
            n480 = local read "rxgain (1-4)"() -> (w1064:i32[])
            n481 = local read "cal_rf_ampl"() -> (w1066:dbl)
            n482 = local read "cal_rf_freq"() -> (w1067:dbl)
            n483 = local read "peak_gain"() -> (w1060:dbl)
            n484 = local read "ob_temp"() -> (w1079:sgl[])
            n485 = local read "ref_freq"() -> (w1089:dbl)
            n486 = local read "fout_bp"() -> (w1084:dbl)
            n487 = Subtract(x=w1097, y=w1096) -> (x-y=w1094:dbl)
            "iteration Time(s)" <- w1094
            n488 = Boolean To (0,1)(Boolean=w1049) -> (0, 1=w1061:i16)
            n489 = local read "if_freq"() -> (w1062:dbl)
            n490 = local read "rdiv(v)"() -> (w1092:dbl[])
            n491 = local read "rdiv(i)"() -> (w1091:dbl[])
            n492 = local read "rx_filt"() -> (w1083:i32)
            n493 = local read "bpf"() -> (w1065:i32)
            n494 = local read "s-n"() -> (w1085:dbl)
            n495 = local read "rdv"() -> (w1093:dbl[])
            n496 = local read "nf"() -> (w1047:dbl)
            n497 = Build Array (concatenate)(w1090, w1083, w1065, w1064, w1089, w1062, w1081, w1060, w1080, w1088, w1086, w1085, w1084, w1047, w1093, w1092, w1091, w1079, w1077, w1067, w1066, w1094, w1095, w1061) -> (w1069:dbl[])
            n498 = for {
              tunnel: w1069 -> [w1099] mode=indexing
              tunnel: [w1098] -> w1068 mode=indexing
              n499 = Format Into String(format string="%#f", initial string="", w1099) -> (resulting string=w1098:string)  [unwired: 1 in, 1 out]
            }
            n500 = Get Date/Time In Seconds() -> (seconds since 1Jan1904=w1075:timestamp)
            n501 = local read "adc#ofresync"() -> (w1052:i32)
            n502 = local read "adc_chan_id"() -> (w1057:string)
            n503 = local read "cal_adc_delay"() -> (w1059:string)
            n504 = local read "adc_lock(t)"() -> (w1054:bool)
            n505 = global read "Test Parameter Globals_1.0.0.vi" "Global SN"() -> (w1076:string)
            n506 = local read "noisecapture path"() -> (w1082:string)
            n507 = local read "sigcapture path"() -> (w1087:string)
            n508 = Get Date/Time String(seconds (now)=w1075, want seconds? (F)=TRUE) -> (date string=w1074:string, time string=w1073:string)  [unwired: 1 in]
            n509 = call <vilib>:"Space Constant.vi"() -> ("String"=w1072:string)
            n510 = local read "adcsync"() -> (w1063:string)
            n511 = Concatenate Strings(w1074, w1072, w1073) -> (w1071:string)
            n512 = call <vilib>:"Trim Whitespace.vi"("string"=w1057, "location (both)"=w1055) -> ("trimmed string"=w1056:string)
            n513 = call <vilib>:"Trim Whitespace.vi"("string"=w1059) -> ("trimmed string"=w1058:string)  [unwired: 1 in]
            n514 = call <vilib>:"Trim Whitespace.vi"("string"=w1076) -> ("trimmed string"=w1078:string)  [unwired: 1 in]
            n515 = Format Into String(format string="%d", w1054) -> (resulting string=w1053:string)  [unwired: 2 in, 1 out]
            n516 = Format Into String(format string="%d", w1052) -> (resulting string=w1050:string)  [unwired: 2 in, 1 out]
          }
        }
        n517 = Unbundle By Name(w77) -> ("status"=w76:bool, "code"=w79:i32, "source"=w72:string)
        n518 = Not(x=w76) -> (.not. x?=w80:bool)
        n519 = Equal To 0?(x=w75) -> (x = 0?=w73:bool)
        n520 = Or(x=w80, y=w83) -> (x .or. y?=w81:bool)
        n521 = And(x=w73, y=w76) -> (x .and. y?=w74:bool)
        n522 = case shown="False" w74 {
          tunnel: w79 -> [_ w126]
          tunnel: [w123 w125] -> w78
          tunnel: w77 -> [w123 w124]
          frame False {
          }
          frame True {
            n523 = call <vilib>:"Clear Errors.vi"("error in (no error)"=w124, "specific error code to clear (0: all)"=w126) -> ("error out"=w125:errorcluster)  [unwired: 4 in, 1 out]
          }
        }
      }
    }
    frame #2 {
      n524 = call <vilib>:"Space Constant.vi"() -> ("String"=w1104:string)
      n525 = flat-sequence {
        tunnel: [w1134] -> w1107
        frame #0 {
          n526 = local read "ps_meas(i)(w)"() -> (w1152:dbl[])
          n527 = local read "MEAS_SNR"() -> (w1141:bool)
          n528 = local read "GAIN_HSL"() -> (w1148:dbl)
          n529 = local read "peak_gain"() -> (w1150:dbl)
          n530 = local read "GAIN_LSL"() -> (w1149:dbl)
          n531 = local read "NF_HSL"() -> (w1147:dbl)
          n532 = local read "NF_LSL"() -> (w1146:dbl)
          n533 = local read "MEAS_PS"() -> (w1142:bool)
          n534 = local read "DC_HSL"() -> (w1154:dbl)
          n535 = local read "DC_LSL"() -> (w1153:dbl)
          n536 = local read "nf"() -> (w1145:dbl)
          n537 = Index Array(array=w1152, index=1) -> (element=w1144:dbl)
          n538 = case shown="False" w1142 {
            tunnel: w1144 -> [_ w1178]
            tunnel: w1154 -> [_ w1177]
            tunnel: w1153 -> [_ w1176]
            tunnel: [w1172 w1175] -> w1140
            tunnel: [w1172 w1174] -> w1139
            tunnel: [TRUE w1173] -> w1132
            frame False {
              w1172 = "-1"
            }
            frame True {
              n539 = Number To Fractional String(number=w1177) -> (F-format string=w1175:string)  [unwired: 3 in]
              n540 = In Range and Coerce(upper limit=w1177, x=w1178, lower limit=w1176) -> (In Range?=w1173:bool)  [unwired: 1 out]
              n541 = Number To Fractional String(number=w1176) -> (F-format string=w1174:string)  [unwired: 3 in]
            }
          }
          n542 = case shown="True" TRUE {
            tunnel: w1150 -> [_ w1170]
            tunnel: w1148 -> [_ w1169]
            tunnel: w1149 -> [_ w1168]
            tunnel: [w1164 w1167] -> w1138
            tunnel: [w1164 w1166] -> w1137
            tunnel: [TRUE w1165] -> w1131
            frame False {
              w1164 = "-1"
            }
            frame True {
              n543 = Number To Fractional String(number=w1169) -> (F-format string=w1167:string)  [unwired: 3 in]
              n544 = In Range and Coerce(upper limit=w1169, x=w1170, lower limit=w1168) -> (In Range?=w1165:bool)  [unwired: 1 out]
              n545 = Number To Fractional String(number=w1168) -> (F-format string=w1166:string)  [unwired: 3 in]
            }
          }
          n546 = case shown="True" w1141 {
            tunnel: w1145 -> [_ w1162]
            tunnel: w1147 -> [_ w1161]
            tunnel: w1146 -> [_ w1160]
            tunnel: [w1156 w1159] -> w1136
            tunnel: [w1156 w1158] -> w1135
            tunnel: [TRUE w1157] -> w1130
            frame False {
              w1156 = "-1"
            }
            frame True {
              n547 = Number To Fractional String(number=w1161) -> (F-format string=w1159:string)  [unwired: 3 in]
              n548 = In Range and Coerce(upper limit=w1161, x=w1162, lower limit=w1160) -> (In Range?=w1157:bool)  [unwired: 1 out]
              n549 = Number To Fractional String(number=w1160) -> (F-format string=w1158:string)  [unwired: 3 in]
            }
          }
          n550 = local read "ps_meas(i)(w)"() -> (w1123:dbl[])
          n551 = local read "peak_gain"() -> (w1121:dbl)
          n552 = Index Array(array=w1123, index=1) -> (element=w1122:dbl)
          n553 = local read "nf"() -> (w1120:dbl)
          n554 = Format Into String(format string="%d%d%d", w1132, w1131, w1130) -> (resulting string=w1133:string)  [unwired: 2 in, 1 out]
          n555 = Build Array(w1132, w1131, w1130) -> (w1129:bool[])
          n556 = And Array Elements(Boolean array=w1129) -> (logical AND=w1128:bool)
          n557 = call "Prod_Screen.vi"("gain_in"=w1121, "nf_in"=w1120, "pow_in"=w1122) -> ("rx_p-f"=w1118:string, "RX-PASS?(T)"=w1124:bool)  [unwired: 11 in, 4 out]
          "RX-PASS?(T)" <- w1124
          n558 = global write "Test Parameter Globals_1.0.0.vi" "Global_Pass(T)"(w1124) -> ()
          n559 = Format Into String(format string="%d", w1128) -> (resulting string=w1126:string)  [unwired: 2 in, 1 out]
          n560 = Build Array(w1140, w1139, w1138, w1137, w1136, w1135, w1133, w1126, w1118) -> (w1134:string[])
        }
      }
      n561 = Array To Spreadsheet String(delimiter (Tab)=w1104, array=w1105, 3:"" ("format string")) -> ()  [unwired: 1 out]
      n562 = local read "readback"() -> (w1102:string)
    }
    frame #3 {
      n563 = local read "result path"() -> (w1179:string)
      n564 = Search and Replace String(replace all?=TRUE ("replace all? (F)"), input string=w1194, search string="\r\n", replace string="" ("replace string (\"\")")) -> (result string=w1195:string)  [unwired: 4 in, 3 out]
      n565 = Insert Into Array(array=w1190, new element #1=w1189, new element #2=w1188, new element #3=w1187, new element #4=w1186, new element #5=w1195, new element #6=w1185, new element #7=w1184, new element #8=w1183, new element #9=w1182, new element #10=w1181, new element #11=w1180, new element #12=w1179) -> (w1197:string[])  [unwired: 1 in]
      n566 = Array Size(array=w1197) -> (size(s)=w1196:i32)
      n567 = for {
        N: w1196 -> [_]
        tunnel: w1197 -> [w1201] mode=indexing
        tunnel: [w1201] -> w1198 mode=indexing if=w1200
        n568 = Empty String/Path?(string/path=w1201) -> (empty?=w1202:bool)
        n569 = Not(x=w1202) -> (.not. x?=w1200:bool)
      }
      "Payload Results" <- w1198
    }
  }
  "error out" <- w17
